vi "ImgRotateCommand.vi"(7 "OutputFiles":path, 8 "Error in":errorcluster caption="Error in (no error)", 11 "ImgPath":path) -> (0 "Error out":errorcluster, 2 "error":bool, 3 "ImgPath out":path)   [LabVIEW 2016, in "EPUB.lvclass"]
uses:
  EPUB.lvclass
panel:
  out "CommandLine":string
  out "standard error":string caption="标准错误"
  out "standard output":string caption="标准输出"
  out "return code":i32 caption="返回代码"
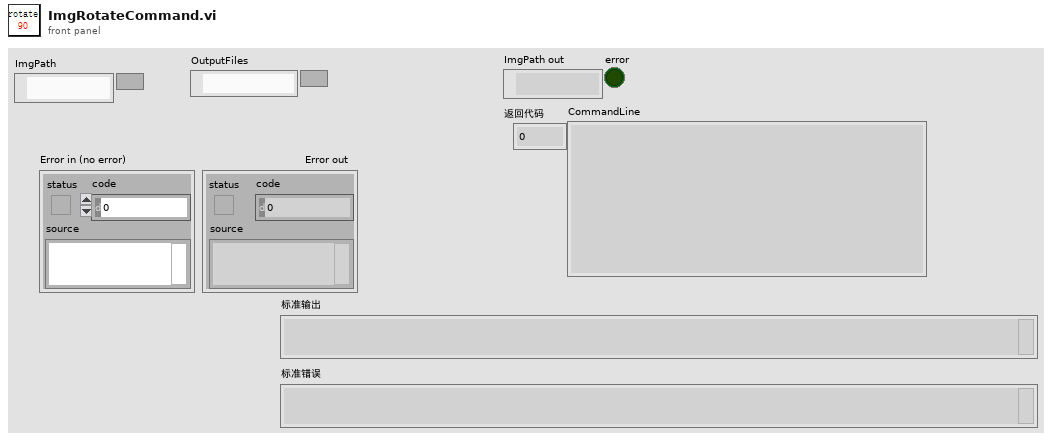
[diagram p1: front panel]
types:
  T1 = cluster{"Enable":bool, "ParaSign":string, "OutputFiles":path[]}
  T2 = cluster{"Enable":bool, "ParaSign":string, "InputFile":path[]}
  T3 = cluster{"Path？":bool, "ComPath":path, "ComText":string}
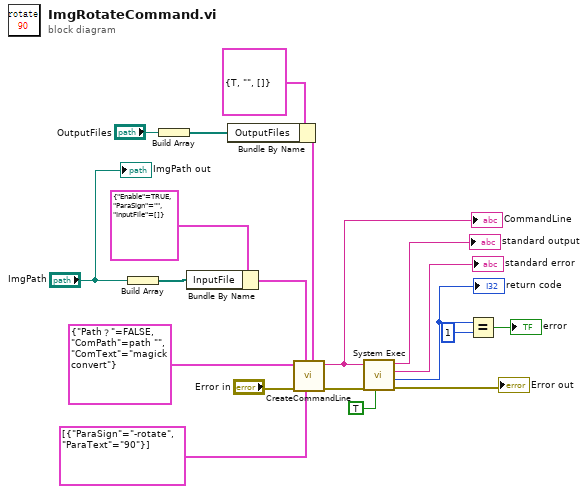
[diagram p0: block diagram]
diagram:
  n1 = Build Array("ImgPath") -> (w17:path[])
  n2 = Build Array("OutputFiles") -> (w1:path[])
  n3 = Bundle By Name(cluster=T2 {"Enable"=TRUE, "ParaSign"="", "InputFile"=[]} ("Input"), "InputFile"=w17) -> (w11:T2)
  n4 = Bundle By Name(cluster=T1 {"Enable"=TRUE, "ParaSign"="", "OutputFiles"=[]} ("Output"), "OutputFiles"=w1) -> (w3:T1)
  n5 = call <vilib>:"CreateCommandLine.vi"("Output"=w3, "ComPara"=cluster{"ParaSign":string, "ParaText":string}[] [{"ParaSign"="-rotate", "ParaText"="90"}], "Input"=w11, "Error in"="Error in", "Command"=T3 {"Path？"=FALSE, "ComPath"=path "", "ComText"="magick convert"}) -> ("Error out"=w15:errorcluster, "CommandLine"=w16:string)  [unwired: 5 in]
  "CommandLine" <- w16
  n6 = call <vilib>:"System Exec.vi"("run minimized? (F)"=TRUE, "error in (no error)"=w15, "command line"=w16) -> ("error out"=→"Error out":errorcluster, "return code"=w7:i32, "standard error"=→"standard error":string, "standard output"=→"standard output":string)  [unwired: 5 in]
  "return code" <- w7
  n7 = Equal?(x=w7, y=1) -> (x = y?=→"error":bool)
  "ImgPath out" <- "ImgPath"
